vi "PH_Cont-601k_PSU.ProcEvents.vi"(0 "i ref in":refnum<vi>, 5 "error in":errorcluster) -> (14 "i ref out":refnum<vi>, 19 "error out":errorcluster)   [LabVIEW 2014, in "PH_Cont-601k_PSU.lvlib"]
doc: "This method is used to define the events the object will listen to. Add your own events here."
uses:
  PH_Cont-601k_PSU.lvlib
  CS_Core/BaseProcess/BaseProcess.event definition.ctl
  CS_Core/CAEObj/CAEObj.event definition.ctl
  CS_Core/BaseProcess/BaseProcess.descriptor string definition.ctl
  CS_Core/BaseProcess/BaseProcess.lvlib
  CS_Core/CAEObj/CAEObj.lvlib
  PH_Basics/PH_Common/PH_Common.lvlib
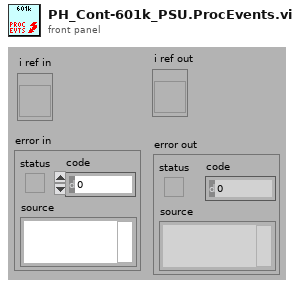
[diagram p1: front panel]
types:
  T1 = typedef "BaseProcess.lvlib/BaseProcess.event definition.ctl" = cluster{"CAEEvtDef":T2, "Data Descriptor":T3}
  T2 = typedef "CAEObj.lvlib/CAEObj.event definition.ctl" = cluster{"URL":string, "enable":bool, "ignoreResID":bool}
  T3 = typedef "BaseProcess.lvlib/BaseProcess.descriptor string definition.ctl" = string
  T4 = typedef "PH_Cont-601k_PSU.lvlib/PH_Cont-601k_PSU.i attribute.ctl" = cluster{"GUI Refs":T5, "Interlock":bool, "Service ID applied Voltage":i32, "Device Settings":cluster{"Configuration":T6, "Flash Interval [s]":dbl, "Mode":T7, "Voltage [V]":u16, "Charge":bool, "VISA resource name":refnum<visa-resource-name>}, "Readyness":T8, "Information":cluster{"VISA resource name":refnum<visa-resource-name>, "Tagname Power On":string, "Interlock":cluster{"Instance":string, "Tagname":string}, "Limits [V]":cluster{"Lower":dbl, "Upper":dbl}, "Tagname PSU On":string}, "R2S":bool, "Charge is allowed":bool}
  T5 = typedef "PH_Cont-601k_PSU.lvlib/PH_Cont-601k_PSU.GUI Refs.ctl" = cluster{"Power On":refnum<vi>, "Hard- and Software":refnum<vi>, "Device Status":refnum<vi>, "Device Error":refnum<vi>, "Configuration":refnum<vi>, "Flash Interval [s]":refnum<vi>, "Interlock":refnum<vi>, "Interlock Indicator":refnum<vi>, "Voltage [V]":refnum<vi>, "Readyness":refnum<vi>, "Mode":refnum<vi>, "Reset Error":refnum<vi>, "Expert working":refnum<vi>, "Charge":refnum<vi>, "PSU On":refnum<vi>}
  T6 = typedef "PH_Cont-601k_PSU.lvlib/PH_Cont-601k_PSU.Configuration.ctl" = u16
  T7 = typedef "PH_Cont-601k_PSU.lvlib/PH_Cont-601k_PSU.Mode.ctl" = enum32{"STOP", "STANDBY", "READY", "EMISSION", "ERROR"}
  T8 = typedef "PH_Cont-601k_PSU.lvlib/PH_Cont-601k_PSU.Readyness.ctl" = cluster{"Program":T9, "Device":T10}
  T9 = typedef "PH_Cont-601k_PSU.lvlib/PH_Cont-601k_PSU.Readyness Program.ctl" = enum32{"OFF", "POWER", "INTERLOCK"}
  T10 = typedef "PH_Cont-601k_PSU.lvlib/PH_Cont-601k_PSU.Readyness Device.ctl" = enum32{"OFF", "CONNECTING", "CONNECTED", "OPERATING", "EOC", "ERROR"}
  T11 = typedef "PH_Common.lvlib/PH_DIM.Event Declarer.ctl" = cluster{"Service Name":string, "Selector":string}
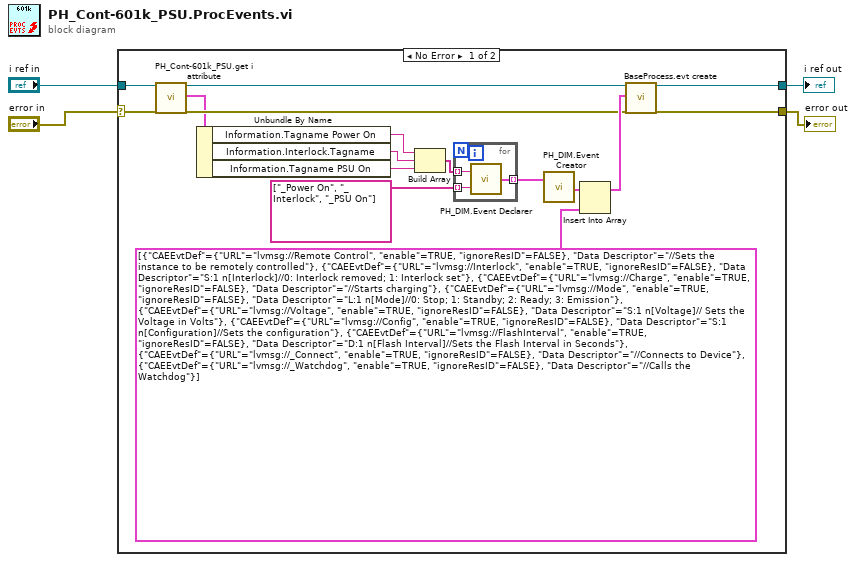
[diagram p0: block diagram]
diagram:
  n1 = case shown="No Error" "error in" {
    selector: "error in" -> [w11 w24]
    tunnel: "i ref in" -> [w10 w25]
    tunnel: [w20 w25] -> w3
    tunnel: [w19 w24] -> w2
    frame No Error {
      n2 = call "PH_Cont-601k_PSU.get i attribute.vi"("i ref in"=w10, "error in (no error)"=w11) -> ("i ref out"=w12:refnum<vi>, "i attribute"=w8:T4, "error out"=w13:errorcluster)  [unwired: 15 in]
      n3 = Unbundle By Name(w8) -> ("Information.Tagname Power On"=w7:string, "Information.Interlock.Tagname"=w6:string, "Information.Tagname PSU On"=w5:string)
      n4 = Build Array(w7, w6, w5) -> (w14:string[])
      n5 = for {
        tunnel: [w21] -> w15 mode=indexing
        tunnel: w14 -> [w23] mode=indexing
        tunnel: string[] ["_Power On", "_Interlock", "_PSU On"] -> [w22] mode=indexing
        n6 = call "PH_DIM.Event Declarer.vi"("Selector"=w22, "Service Name"=w23) -> ("declared DIM Event"=w21:T11)
      }
      n7 = call "PH_DIM.Event Creator.vi"("Trendmessage Services"=w15) -> ("DIM Service Events"=w16:T1[])  [unwired: 18 in]
      n8 = Insert Into Array(array=w16, new element=T1[] [{"CAEEvtDef"={"URL"="lvmsg://Remote Control", "enable"=TRUE, "ignoreResID"=FALSE}, "Data Descriptor"="//Sets the instance to be remotely controlled"}, {"CAEEvtDef"={"URL"="lvmsg://Interlock", "enable"=TRUE, "ignoreResID"=FALSE}, "Data Descriptor"="S:1 n[Interlock]//0: Interlock removed; 1: Interlock set"}, {"CAEEvtDef"={"URL"="lvmsg://Charge", "enable"=TRUE, "ignoreResID"=FALSE}, "Data Descriptor"="//Starts charging"}, {"CAEEvtDef"={"URL"="lvmsg://Mode", "enable"=TRUE, "ignoreResID"=FALSE}, "Data Descriptor"="L:1 n[Mode]//0: Stop; 1: Standby; 2: Ready; 3: Emission"}, {"CAEEvtDef"={"URL"="lvmsg://Voltage", "enable"=TRUE, "ignoreResID"=FALSE}, "Data Descriptor"="S:1 n[Voltage]// Sets the Voltage in Volts"}, {"CAEEvtDef"={"URL"="lvmsg://Config", "enable"=TRUE, "ignoreResID"=FALSE}, "Data Descriptor"="S:1 n[Configuration]//Sets the configuration"}, {"CAEEvtDef"={"URL"="lvmsg://FlashInterval", "enable"=TRUE, "ignoreResID"=FALSE}, "Data Descriptor"="D:1 n[Flash Interval]//Sets the Flash Interval in Seconds"}, {"CAEEvtDef"={"URL"="lvmsg://_Connect", "enable"=TRUE, "ignoreResID"=FALSE}, "Data Descriptor"="//Connects to Device"}, {"CAEEvtDef"={"URL"="lvmsg://_Watchdog", "enable"=TRUE, "ignoreResID"=FALSE}, "Data Descriptor"="//Calls the Watchdog"}] ("new events")) -> (w18:T1[])  [unwired: 1 in]
      n9 = call "BaseProcess.evt create.vi"("i ref in"=w12, "newEvents"=w18, "error in (no error)"=w13) -> ("i ref out"=w20:refnum<vi>, "error out"=w19:errorcluster)  [unwired: 13 in, 2 out]
    }
    frame Error {
    }
  }
  "i ref out" <- w3
  "error out" <- w2
